vi "Main.Constants.vi"() -> ()   [LabVIEW 2015, in "Single Station Execution.lvlib"]
uses:
  Single Station Execution.lvlib
  <vilib>/Utility/miscctls.llb/LVBoundsTypeDef.ctl
  Types/Sequence.Reference.ctl
panel:
  in  "Execution.SaveMenuTag":string="Config.Save"
  in  "Execution.LoadConfigTag":string="Config.Load"
  in  "Waveform.LocalSuffix":string="_Array"
  in  "XML.RestartVersion":string="1.0.0"
  in  "XML.RestartVersionTag":string="RestartVersion"
  in  "XML.SSEVersion":string="1.0.0"
  in  "XML.SSEVersionTag":string="SSEVersion"
  in  "Sequence.StartTime":string="StartTime"
  in  "Task.Duration":string="Duration"
  in  "Sequence.StartingDuration":string="SequenceStartingDuration"
  in  "LinerSweptSine.Syntax":string="lSin (Bias, Amp, StartHz, EndHz)"
  in  "ForcedRamp.Syntax":string="fRamp (StartVal, EndVal)"
  in  "SweptSine.LocalSuffix":string="_Array"
  in  "SweptSine.GenRateHz":dbl=1000.0
  in  "LogSweptSine.Syntax":string="eSin (Bias, Amp, StartHz, EndHz)"
  in  "Sine.Syntax":string="Sin (Bias, Amp, Hz)"
  in  "Execution.RestartMenuTag":string="App.Restart"
  in  "Execution.NewMenuTag":string="App.New"
  in  "INI.FileName":string="Settings.INI"
  in  "Task.StepManagePrefix":string="StepManage_"
  in  "Task.StepExePrefix":string="StepExe_"
  in  "Sequence.ForLoopBaseVar":string="i"
  in  "Task.Abort":string="Abort"
  in  "Task.Sequence":string="Sequence"
  in  "Sequence.TempStepInfo":string="TempStepInfo"
  in  "Sequence.StartingStep":string="SequenceStartingStep"
  in  "Sequence.StartingIteration":string="SequenceStartingIteration"
  in  "References":T1[](array[typedef])=[{"Name"="Ramp", "RelativePath"="\\nivs.lib\\Sequence Library\\Standard\\Waveforms\\Ramp.nivsseq"}, {"Name"="Wait", "RelativePath"="\\nivs.lib\\Sequence Library\\Standard\\Timing\\Wait.nivsseq"}, {"Name"="SineWave", "RelativePath"="\\nivs.lib\\Sequence Library\\Standard\\Waveforms\\SineWave.nivsseq"}, {"Name"="PlayWaveform", "RelativePath"="\\nivs.lib\\Sequence Library\\Standard\\Waveforms\\PlayWaveform.nivsseq"}, {"Name"="WaitUntilSettled", "RelativePath"="\\nivs.lib\\Sequence Library\\Standard\\Timing\\WaitUntilSettled.nivsseq"}]
  in  "Sequence.NewChannelSize":T2={"Width"=175, "Height"=0}
  in  "Sequence.BaseHeaderSize":T2[](array[typedef])=[{"Width"=81, "Height"=0}, {"Width"=56, "Height"=0}, {"Width"=300, "Height"=0}, {"Width"=175, "Height"=0}]
  in  "Sequence.BaseHeader":string[](array[string])=["Step\nDuration (secs)", "Operator", "Additional Condition(s)"]
  in  "iStep.Syntax":string="iStep (StartVal, EndVal, StepVal)"
  in  "Menu.PropertyPrefix":string="Property."
  in  "Menu.ConditionsPrefix":string="Conditions."
  in  "NoChange.Syntax":string="Unchanged"
  in  "Menu.StepPrefix":string="Step."
  in  "Ramp.Syntax":string="Ramp (EndVal)"
  in  "Step.Syntax":string="Step (Val)"
  in  "# of Static Columns":u32=3
  in  "Menu.ChannelPrefix":string="Channel."
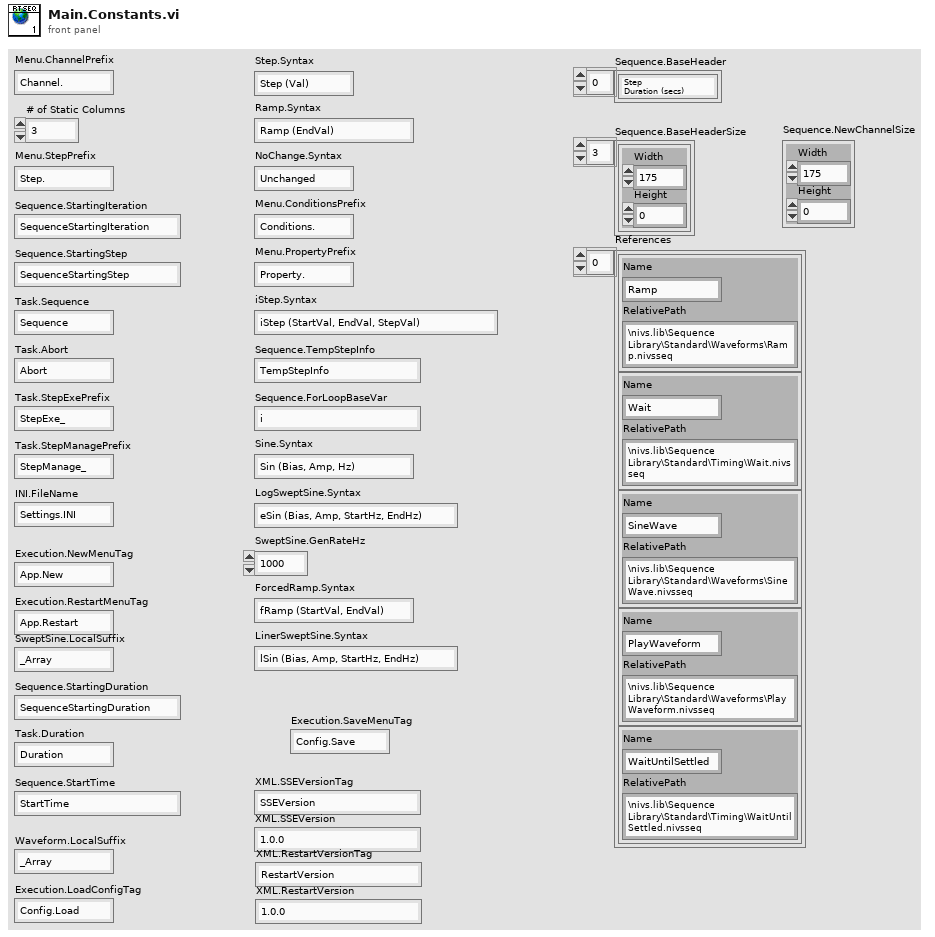
[diagram p1: front panel]
types:
  T1 = typedef "Single Station Execution.lvlib/Sequence.Reference.ctl" = cluster{"Name":string, "RelativePath":string}
  T2 = typedef "LVBoundsTypeDef.ctl" = cluster{"Width":u32, "Height":u32}
diagram:
